vi "Create Cow.vi"() -> (3 "Cow.lvclass":refnum<class "Cow.lvclass">)   [LabVIEW 2018, in "Cow.lvclass"]
uses:
  Cow.lvclass
  animal/Animal.lvclass
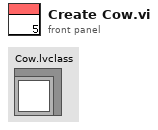
[diagram p1: front panel]
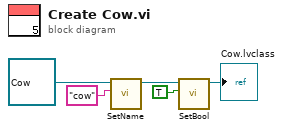
[diagram p0: block diagram]
diagram:
  n1 = call "SetName.vi"("Name"="cow", "Animal in"=refnum<class "Cow.lvclass"> refnum ("Cow.lvclass")) -> ("Animal out"=w3:refnum<class "Cow.lvclass">)  [unwired: 8 in, 1 out]
  n2 = call "SetBool.vi"("Bool"=TRUE, "Animal in"=w3) -> ("Animal out"=→"Cow.lvclass":refnum<class "Cow.lvclass">)  [unwired: 8 in, 1 out]
